vi "SP Coerce CH Controls.vi"(4 "Parameters Measured":T1[](array[typedef]) {"Channel" min=1 max=99 step=1; "Parameter"."Stimulus Port" min=1 step=1; "Parameter"."Response Port" min=1 step=1}, 5 "Formatted Data?":bool, 7 "CH Controls In":T5[](array[typedef])=[{"Trace Orientation"=enum."Overlay", "Frequency"={"Change Frequency"=FALSE, "Start"=500.0, "Stop"=1500.0, "Units"=enum."MHz"}, "Markers"=[], "Traces"=[]}, {"Trace Orientation"=enum."Overlay", "Frequency"={"Change Frequency"=FALSE, "Start"=500.0, "Stop"=1500.0, "Units"=enum."MHz"}, "Markers"=[], "Traces"=[]}, {"Trace Orientation"=enum."Overlay", "Frequency"={"Change Frequency"=FALSE, "Start"=500.0, "Stop"=1500.0, "Units"=enum."MHz"}, "Markers"=[], "Traces"=[]}, {"Trace Orientation"=enum."Overlay", "Frequency"={"Change Frequency"=FALSE, "Start"=500.0, "Stop"=1500.0, "Units"=enum."MHz"}, "Markers"=[], "Traces"=[]}] {"Traces"."Reference" format="%#.2g"; "Traces"."Display Data" items=["Data", "Memory", "Data/Memory"]; "Traces"."Format" items=["Log Mag", "Phase", "Expanded Phase", "Delay", "Smith", "Polar", "Lin Mag", "SWR", "Loss", "Real", "Imaginary"]; "Traces"."Scale" min=0.001 step=1.0 format="%#.2g"; "Traces"."Position" min=0.0 max=10.0; "Frequency"."Stop" format="%.3g"; "Frequency"."Start" format="%.3g"}) -> (1 "CH Controls Out":T5[](array[typedef])=[{"Trace Orientation"=enum."Overlay", "Frequency"={"Change Frequency"=FALSE, "Start"=500.0, "Stop"=1500.0, "Units"=enum."MHz"}, "Markers"=[], "Traces"=[]}, {"Trace Orientation"=enum."Overlay", "Frequency"={"Change Frequency"=FALSE, "Start"=500.0, "Stop"=1500.0, "Units"=enum."MHz"}, "Markers"=[], "Traces"=[]}, {"Trace Orientation"=enum."Overlay", "Frequency"={"Change Frequency"=FALSE, "Start"=500.0, "Stop"=1500.0, "Units"=enum."MHz"}, "Markers"=[], "Traces"=[]}, {"Trace Orientation"=enum."Overlay", "Frequency"={"Change Frequency"=FALSE, "Start"=500.0, "Stop"=1500.0, "Units"=enum."MHz"}, "Markers"=[], "Traces"=[]}] {"Traces"."Reference" format="%#.2g"; "Traces"."Display Data" items=["Data", "Memory", "Data/Memory"]; "Traces"."Format" items=["Log Mag", "Phase", "Expanded Phase", "Delay", "Smith", "Polar", "Lin Mag", "SWR", "Loss", "Real", "Imaginary"]; "Traces"."Scale" min=0.001 step=1.0 format="%#.2g"; "Traces"."Position" min=0.0 max=10.0; "Frequency"."Stop" format="%.3g"; "Frequency"."Start" format="%.3g"})   [LabVIEW 2011]
uses:
  TypeDefs/SP Display Plot Controls Cluster.ctl
  TypeDefs/SP Frequency Units.ctl
  TypeDefs/SP Marker Cluster.ctl
  TypeDefs/SP Marker Type.ctl
  TypeDefs/SP Display Trace Controls.ctl
  TypeDefs/SP Display Format.ctl
  TypeDefs/SP Display Data.ctl
  TypeDefs/SP Parameter to Measure.ctl
  TypeDefs/SP Parameter.ctl
  TypeDefs/SP Calibration State.ctl
  TypeDefs/SP Measurement Format.ctl
panel:
  # "Div"
  # "Div"
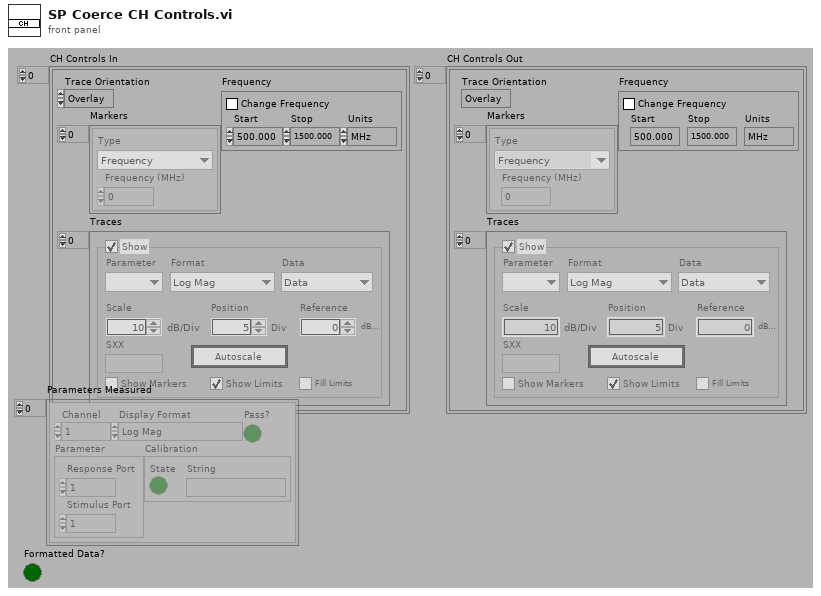
[diagram p1: front panel]
types:
  T1 = typedef "SP Parameter to Measure.ctl" = cluster{"Channel":i8, "Parameter":T2, "Calibration":T3, "Display Format":T4, "Pass?":bool}
  T2 = typedef "SP Parameter.ctl" = cluster{"Stimulus Port":i8, "Response Port":i8}
  T3 = typedef "SP Calibration State.ctl" = cluster{"State":bool, "String":string}
  T4 = typedef "SP Measurement Format.ctl" = enum32{"Log Mag", "Phase", "Delay", "Smith (R+jX)", "Polar (Re/Im)", "Linear Mag", "SWR", "Real", "Imaginary", "Smith (Lin/Phase)", "Smith (Log/Phase)", "Smith (Real/Imag)", "Smith (G+jB)", "Polar (Lin/Phase)", "Polar (Log/Phase)", "Expanded Phase", "Positive Phase", "Inverted Smith", "Unwrapped Phase", "Power Out", "Power In", "Linear Mag/Phase", "Log Mag/Phase", "Real/Imaginary"}
  T5 = typedef "SP Display Plot Controls Cluster.ctl" = cluster{"Trace Orientation":enum32{"Overlay", "Split"}, "Frequency":cluster{"Change Frequency":bool, "Start":dbl, "Stop":dbl, "Units":T6}, "Markers":T7[], "Traces":T9[]}
  T6 = typedef "SP Frequency Units.ctl" = enum16{"Hz", "kHz", "MHz", "GHz", "Points"}
  T7 = typedef "SP Marker Cluster.ctl" = cluster{"Type":T8, "Frequency (MHz)":dbl}
  T8 = typedef "SP Marker Type.ctl" = enum16{"Frequency", "Trace Maximum", "Trace Minimum", "Limit Maximum", "Limit Minimum"}
  T9 = typedef "SP Display Trace Controls.ctl" = cluster{"Trace On":bool, "Measure":i32, "Format":T10, "Autoscale":bool, "Reference":dbl, "\nRefUnit":string, "Position":dbl, "Scale":dbl, "ScaleUnit":string, "LimitOn":bool, "LimitFill":bool, "Display Data":T11, "Show Markers":bool, "SXX":string}
  T10 = typedef "SP Display Format.ctl" = i32
  T11 = typedef "SP Display Data.ctl" = u16
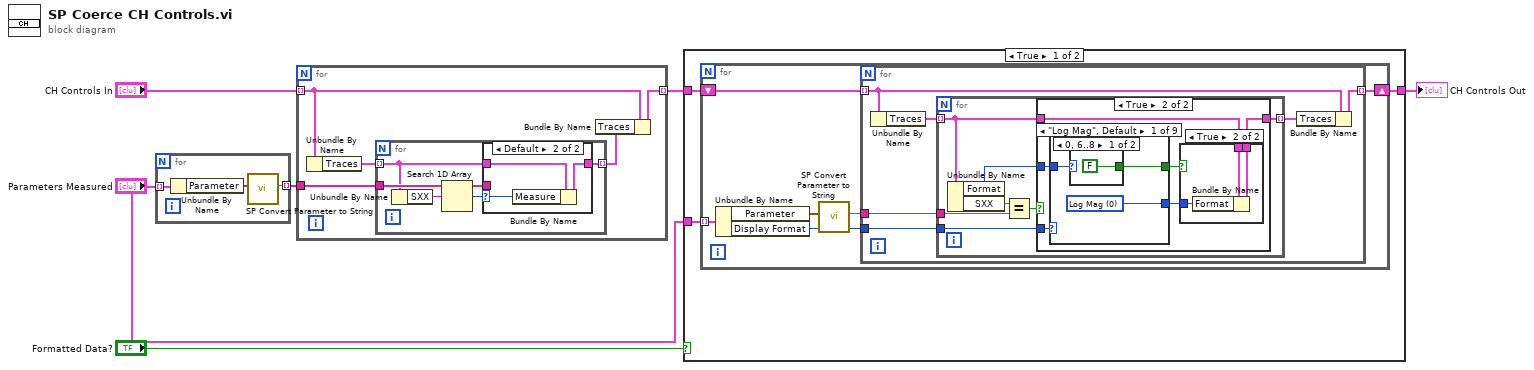
[diagram p0: block diagram]
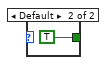
[diagram p4: hidden frame]
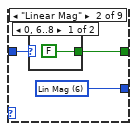
[diagram p5: hidden frame]
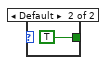
[diagram p6: hidden frame]
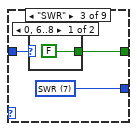
[diagram p7: hidden frame]
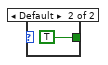
[diagram p8: hidden frame]
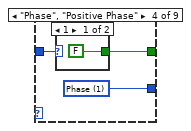
[diagram p9: hidden frame]
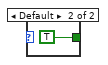
[diagram p10: hidden frame]
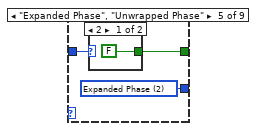
[diagram p11: hidden frame]
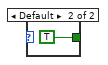
[diagram p12: hidden frame]
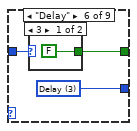
[diagram p13: hidden frame]
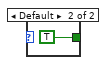
[diagram p14: hidden frame]
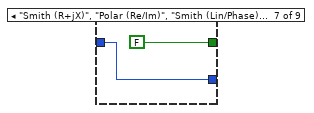
[diagram p15: hidden frame]
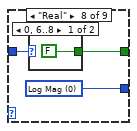
[diagram p16: hidden frame]
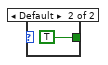
[diagram p17: hidden frame]
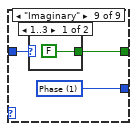
[diagram p18: hidden frame]
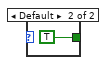
[diagram p19: hidden frame]
diagram:
  n1 = for {
    tunnel: "Parameters Measured" -> [w9] mode=indexing
    tunnel: [w7] -> w6 mode=indexing
    n2 = Unbundle By Name(w9) -> ("Parameter"=w8:T2)
    n3 = call "SP Convert Parameter to String.vi"("Parameter"=w8) -> ("Parameter String"=w7:string)  [unwired: 10 out]
  }
  n4 = for {
    tunnel: "CH Controls In" -> [w12] mode=indexing
    tunnel: [w11] -> w4 mode=indexing
    tunnel: w6 -> [w14]
    n5 = Unbundle By Name(w12) -> ("Traces"=w13:T9[])
    n6 = for {
      tunnel: [w19] -> w10 mode=indexing
      tunnel: w14 -> [w17]
      tunnel: w13 -> [w15] mode=indexing
      n7 = Unbundle By Name(w15) -> ("SXX"=w16:string)
      n8 = Search 1D Array(1D array=w17, element=w16) -> (index of element=w18:i32)  [unwired: 1 out]
      n9 = case shown="Default" w18 {
        selector: w18 -> [_ w23]
        tunnel: w15 -> [w22 w25]
        tunnel: [w21 w24] -> w19
        tunnel: w17 -> [_ _]
        frame -1 {
          n10 = Bundle By Name(cluster=w22, "Measure"=0 ("CH2Control.Measure")) -> (w21:T9)
        }
        frame Default {
          n11 = Bundle By Name(cluster=w25, "Measure"=w23) -> (w24:T9)
        }
      }
    }
    n12 = Bundle By Name(cluster=w12, "Traces"=w10) -> (w11:T5)
  }
  n13 = case shown="True" "Formatted Data?" {
    tunnel: "Parameters Measured" -> [w28 _]
    tunnel: w4 -> [w27 w101]
    tunnel: [w26 w101] -> w1
    frame True {
      n14 = for {
        tunnel: w28 -> [w33] mode=indexing
        shift-right: [w31] -> w26
        shift-left: w27 -> [w34]
        n15 = Unbundle By Name(w33) -> ("Parameter"=w30:T2, "Display Format"=w32:T4)
        n16 = call "SP Convert Parameter to String.vi"("Parameter"=w30) -> ("Parameter String"=w29:string)  [unwired: 10 out]
        n17 = for {
          tunnel: w34 -> [w38] mode=indexing
          tunnel: w29 -> [w40]
          tunnel: w32 -> [w39]
          tunnel: [w37] -> w31 mode=indexing
          n18 = Unbundle By Name(w38) -> ("Traces"=w35:T9[])
          n19 = for {
            tunnel: w40 -> [w47]
            tunnel: w35 -> [w45] mode=indexing
            tunnel: w39 -> [w43]
            tunnel: [w41] -> w36 mode=indexing
            n20 = Unbundle By Name(w45) -> ("Format"=w44:T10, "SXX"=w42:string)
            n21 = Equal?(x=w42, y=w47) -> (x = y?=w46:bool)
            n22 = case shown="True" w46 {
              tunnel: w45 -> [w48 w54]
              tunnel: [w48 w53] -> w41
              tunnel: w44 -> [_ w52]
              tunnel: w43 -> [_ w51]
              frame False {
              }
              frame True {
                n23 = case shown="\"Log Mag\", Default" w51 {
                  tunnel: [w61 w66 w71 w76 w81 w86 w89 w93 w98] -> w50
                  tunnel: w52 -> [w60 w65 w70 w75 w80 w85 w89 w92 w97]
                  tunnel: [w59 w64 w69 w74 w79 w84 FALSE w91 w96] -> w49
                  frame "Log Mag", Default {
                    w61 = T10 0 items=["Log Mag", "Phase", "Expanded Phase", "Delay", "Smith", "Polar", "Lin Mag", "SWR", "Loss", "Real", "Imaginary"] ("Format")
                    n24 = case shown="0, 6..8" w60 {
                      tunnel: [FALSE TRUE] -> w59
                      frame 0, 6..8 {
                      }
                      frame Default {
                      }
                    }
                  }
                  frame "Linear Mag" {
                    w66 = T10 6 items=["Log Mag", "Phase", "Expanded Phase", "Delay", "Smith", "Polar", "Lin Mag", "SWR", "Loss", "Real", "Imaginary"] ("Format")
                    n25 = case shown="0, 6..8" w65 {
                      tunnel: [FALSE TRUE] -> w64
                      frame 0, 6..8 {
                      }
                      frame Default {
                      }
                    }
                  }
                  frame "SWR" {
                    w71 = T10 7 items=["Log Mag", "Phase", "Expanded Phase", "Delay", "Smith", "Polar", "Lin Mag", "SWR", "Loss", "Real", "Imaginary"] ("Format")
                    n26 = case shown="0, 6..8" w70 {
                      tunnel: [FALSE TRUE] -> w69
                      frame 0, 6..8 {
                      }
                      frame Default {
                      }
                    }
                  }
                  frame "Phase", "Positive Phase" {
                    w76 = T10 1 items=["Log Mag", "Phase", "Expanded Phase", "Delay", "Smith", "Polar", "Lin Mag", "SWR", "Loss", "Real", "Imaginary"] ("Format")
                    n27 = case shown="1" w75 {
                      tunnel: [FALSE TRUE] -> w74
                      frame 1 {
                      }
                      frame Default {
                      }
                    }
                  }
                  frame "Expanded Phase", "Unwrapped Phase" {
                    w81 = T10 2 items=["Log Mag", "Phase", "Expanded Phase", "Delay", "Smith", "Polar", "Lin Mag", "SWR", "Loss", "Real", "Imaginary"] ("Format")
                    n28 = case shown="2" w80 {
                      tunnel: [FALSE TRUE] -> w79
                      frame 2 {
                      }
                      frame Default {
                      }
                    }
                  }
                  frame "Delay" {
                    w86 = T10 3 items=["Log Mag", "Phase", "Expanded Phase", "Delay", "Smith", "Polar", "Lin Mag", "SWR", "Loss", "Real", "Imaginary"] ("Format")
                    n29 = case shown="3" w85 {
                      tunnel: [FALSE TRUE] -> w84
                      frame 3 {
                      }
                      frame Default {
                      }
                    }
                  }
                  frame "Smith (R+jX)", "Polar (Re/Im)", "Smith (Lin/Phase)".."Polar (Log/Phase)", "Inverted Smith", "Power Out" {
                  }
                  frame "Real" {
                    w93 = T10 0 items=["Log Mag", "Phase", "Expanded Phase", "Delay", "Smith", "Polar", "Lin Mag", "SWR", "Loss", "Real", "Imaginary"] ("Format")
                    n30 = case shown="0, 6..8" w92 {
                      tunnel: [FALSE TRUE] -> w91
                      frame 0, 6..8 {
                      }
                      frame Default {
                      }
                    }
                  }
                  frame "Imaginary" {
                    w98 = T10 1 items=["Log Mag", "Phase", "Expanded Phase", "Delay", "Smith", "Polar", "Lin Mag", "SWR", "Loss", "Real", "Imaginary"] ("Format")
                    n31 = case shown="1..3" w97 {
                      tunnel: [FALSE TRUE] -> w96
                      frame 1..3 {
                      }
                      frame Default {
                      }
                    }
                  }
                }
                n32 = case shown="True" w49 {
                  tunnel: w54 -> [w55 w58]
                  tunnel: [w55 w57] -> w53
                  tunnel: w50 -> [_ w56]
                  frame False {
                  }
                  frame True {
                    n33 = Bundle By Name(cluster=w58, "Format"=w56) -> (w57:T9)
                  }
                }
              }
            }
          }
          n34 = Bundle By Name(cluster=w38, "Traces"=w36) -> (w37:T5)
        }
      }
    }
    frame False {
    }
  }
  "CH Controls Out" <- w1
